vi "SaveTSVFile.vi"(8 "Task":enum16{"Save Magnitude", "Save Complex"}(ring), 9 "type":enum16{"tsv", "csv"}(ring), 10 "FRF":cluster{"t0":dbl, "dt":dbl, "Y":cdb[]}, 11 "Path":path) -> (0 "error out":errorcluster)   [LabVIEW 2022 SP3]
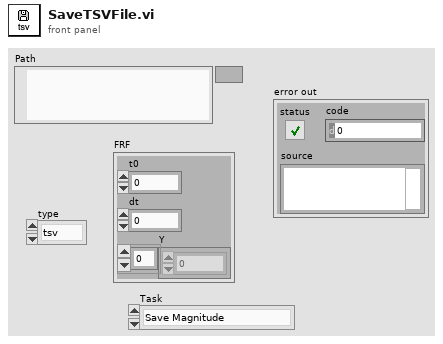
[diagram p1: front panel]
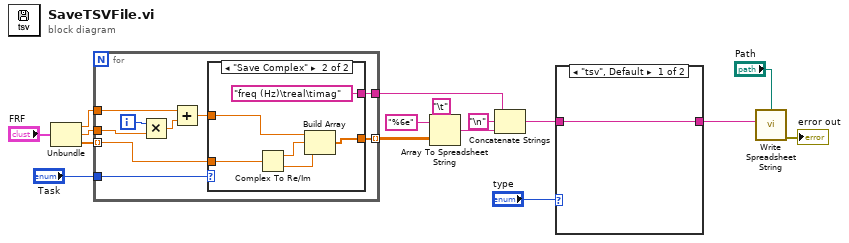
[diagram p0: block diagram]
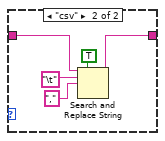
[diagram p2: hidden frame]
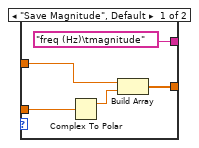
[diagram p3: hidden frame]
diagram:
  n1 = Unbundle("FRF") -> ("t0"=w14:dbl, "dt"=w15:dbl, "Y"=w13:cdb[])
  n2 = for {
    tunnel: w15 -> [w24]
    tunnel: w14 -> [w22]
    tunnel: w13 -> [w20] mode=indexing
    tunnel: [w19] -> w12 mode=indexing
    tunnel: "Task" -> [w18]
    tunnel: [w17] -> w5
    i -> [w23]
    n3 = Multiply(x=w23, y=w24) -> (x*y=w25:dbl)
    n4 = Add(x=w22, y=w25) -> (x+y=w21:dbl)
    n5 = case shown="\"Save Complex\"" w18 {
      tunnel: w21 -> [w30 w36]
      tunnel: w20 -> [w29 w35]
      tunnel: [w28 w34] -> w19
      tunnel: ["freq (Hz)\tmagnitude" ("delimiter (Tab)") "freq (Hz)\treal\timag" ("delimiter (Tab)")] -> w17
      frame "Save Magnitude", Default {
        n6 = Complex To Polar(r * e^(i*theta)=w29) -> (r=w27:dbl)  [unwired: 1 out]
        n7 = Build Array(w30, w27) -> (w28:dbl[])
      }
      frame "Save Complex" {
        n8 = Complex To Re/Im(x + iy=w35) -> (x=w33:dbl, y=w32:dbl)
        n9 = Build Array(w36, w33, w32) -> (w34:dbl[])
      }
    }
  }
  n10 = Array To Spreadsheet String(delimiter (Tab)="\t", array=w12, 3:"%6e" ("format string")) -> (spreadsheet string=w6:string)
  n11 = Concatenate Strings(w5, "\n" ("string"), w6) -> (w3:string)
  n12 = case shown="\"tsv\", Default" "type" {
    tunnel: w3 -> [w37 w42]
    tunnel: [w37 w38] -> w1
    frame "tsv", Default {
    }
    frame "csv" {
      n13 = Search and Replace String(replace all?=TRUE ("replace all? (F)"), input string=w42, search string="\t" ("delimiter (Tab)"), replace string="," ("delimiter (Tab)")) -> (result string=w38:string)  [unwired: 4 in, 3 out]
    }
  }
  n14 = call <vilib>:"Write Spreadsheet String.vi"("spreadsheet string"=w1, "file path (dialog if empty)"="Path") -> ("error out"=→"error out":errorcluster)  [unwired: 8 in, 1 out]
